vi "dvp Vi Get Config String.vi"(6 "pIndex":u32, 7 "unSize":u32, 9 "pszValue":string, 10 "pszName":string, 11 "handle":u32) -> (1 "pszValue out":string, 2 "pszName out":string, 3 "function return":u32(ring), 4 "pIndex out":u32)   [LabVIEW 2018, in "LabViewDVPCamera.lvlib"]
doc: "LabviewDvp2Api dvpStatus dvpViGetConfigString(dvpHandle handle,char *pszName,char *pszValue,dvpUint32 unSize,dvpUint32 *pIndex);"
uses:
  LabViewDVPCamera.lvlib
  LabViewDVPCamera/LabViewDVPCamera.dll
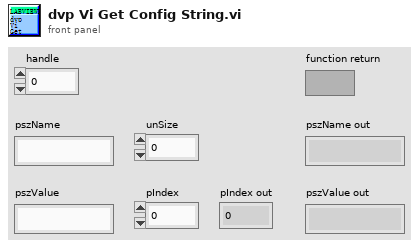
[diagram p1: front panel]
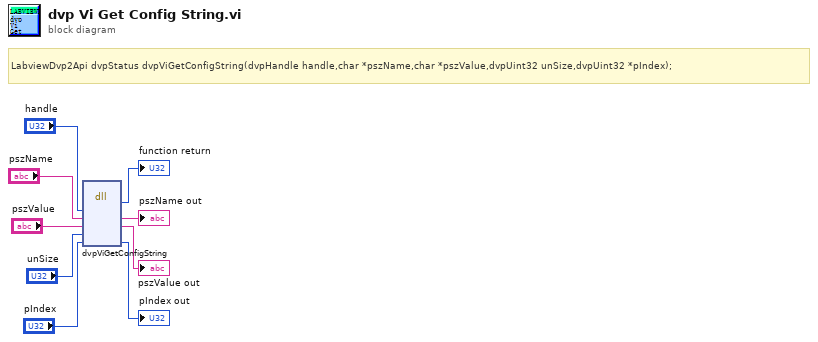
[diagram p0: block diagram]
diagram:
  # "LabviewDvp2Api dvpStatus dvpViGetConfigString(dvpHandle handle,char *pszName,char *pszValue,dvpUint32 unSize,dvpUint32 *pIndex);"
  n1 = dll-call lib="C:/Program Files (x86)/DVP2 Labview cn 64/Sample/LabViewDVPCamera/LabViewDVPCamera.*" fn="dvpViGetConfigString"("handle"="handle", "pszName"="pszName", "pszValue"="pszValue", "unSize"="unSize", "pIndex"="pIndex") -> (→"function return":u32, "pszName"=→"pszName out":string, "pszValue"=→"pszValue out":string, "pIndex"=→"pIndex out":u32)  [unwired: 5 in, 2 out]
